vi "Sscard屏幕.vi"() -> ()   [LabVIEW 2015]
uses:
  Controls Type/square.ctl
  <userlib>/QMH/Message Queue/Support/Message Cluster.ctl
  Global control/global-1.vi
  Global control/global-opc.vi
  <userlib>/QMH/Message Queue/Support/Enqueue Message (Single).vi
  <userlib>/QMH/Message Queue/Support/Enqueue Message (Array).vi
  Global control/global-2.vi
  <userlib>/QMH/User Event - Stop/User Event - Stop.lvlib
  <userlib>/QMH/Message Queue/Message Queue.lvlib
panel:
  in  "70":T1
  in  "60":T1
  out "整流柜远程/本地":enum16{"零位", "本地", "远方"}(ring)
  out "直流继保远程/本地":enum16{"零位", "本地", "远方"}(ring)
  out "上网柜远程/本地":enum16{"零位", "本地", "远方"}(ring)
  out "负极柜远程/本地":enum16{"零位", "本地", "远方"}(ring)
  out "馈线柜远程/本地":enum16{"零位", "本地", "远方"}(ring)
  out "进线柜远程/本地":enum16{"零位", "本地", "远方"}(ring)
  out "整流柜远程/本地":enum16{"零位", "本地", "远方"}(ring)
  out "拉伸界面":bool
  in  "HostThread":variant
  in  "Exit":bool
  out "安全运行":string caption="天"
  out "时间":string="14 : 47 : 23" caption="天"
  out "星期":string caption="星\n期"
  out "日":string caption="天"
  out "月":string caption="天"
  out "年":string caption="天"
  in  "405":T1
  in  "406":T1
  in  "407":T1
  in  "445":T1
  in  "213":T1
  in  "211":T1
  in  "90":T1
  in  "214":T1
  in  "212":T1
  in  "402":T1
  in  "401":T1
  in  "241":T1
  in  "226":T1
  in  "202":T1
  in  "245":T1
  in  "231":T1
  in  "237":bool
  in  "236":bool
  in  "225":bool
  in  "201":bool
  in  "2120":bool
  in  "2130":bool
  in  "2110":bool
  in  "2140":bool
  in  "2121":bool
  in  "2124":bool
  in  "2141":bool
  in  "2113":bool
  in  "2111":bool
  in  "2131":bool
  in  "404":bool
  in  "75":bool
  in  "65":bool
  in  "2451":bool
  in  "241-7":bool
  in  "231-7":bool
  in  "237-7":bool
  in  "236-7":bool
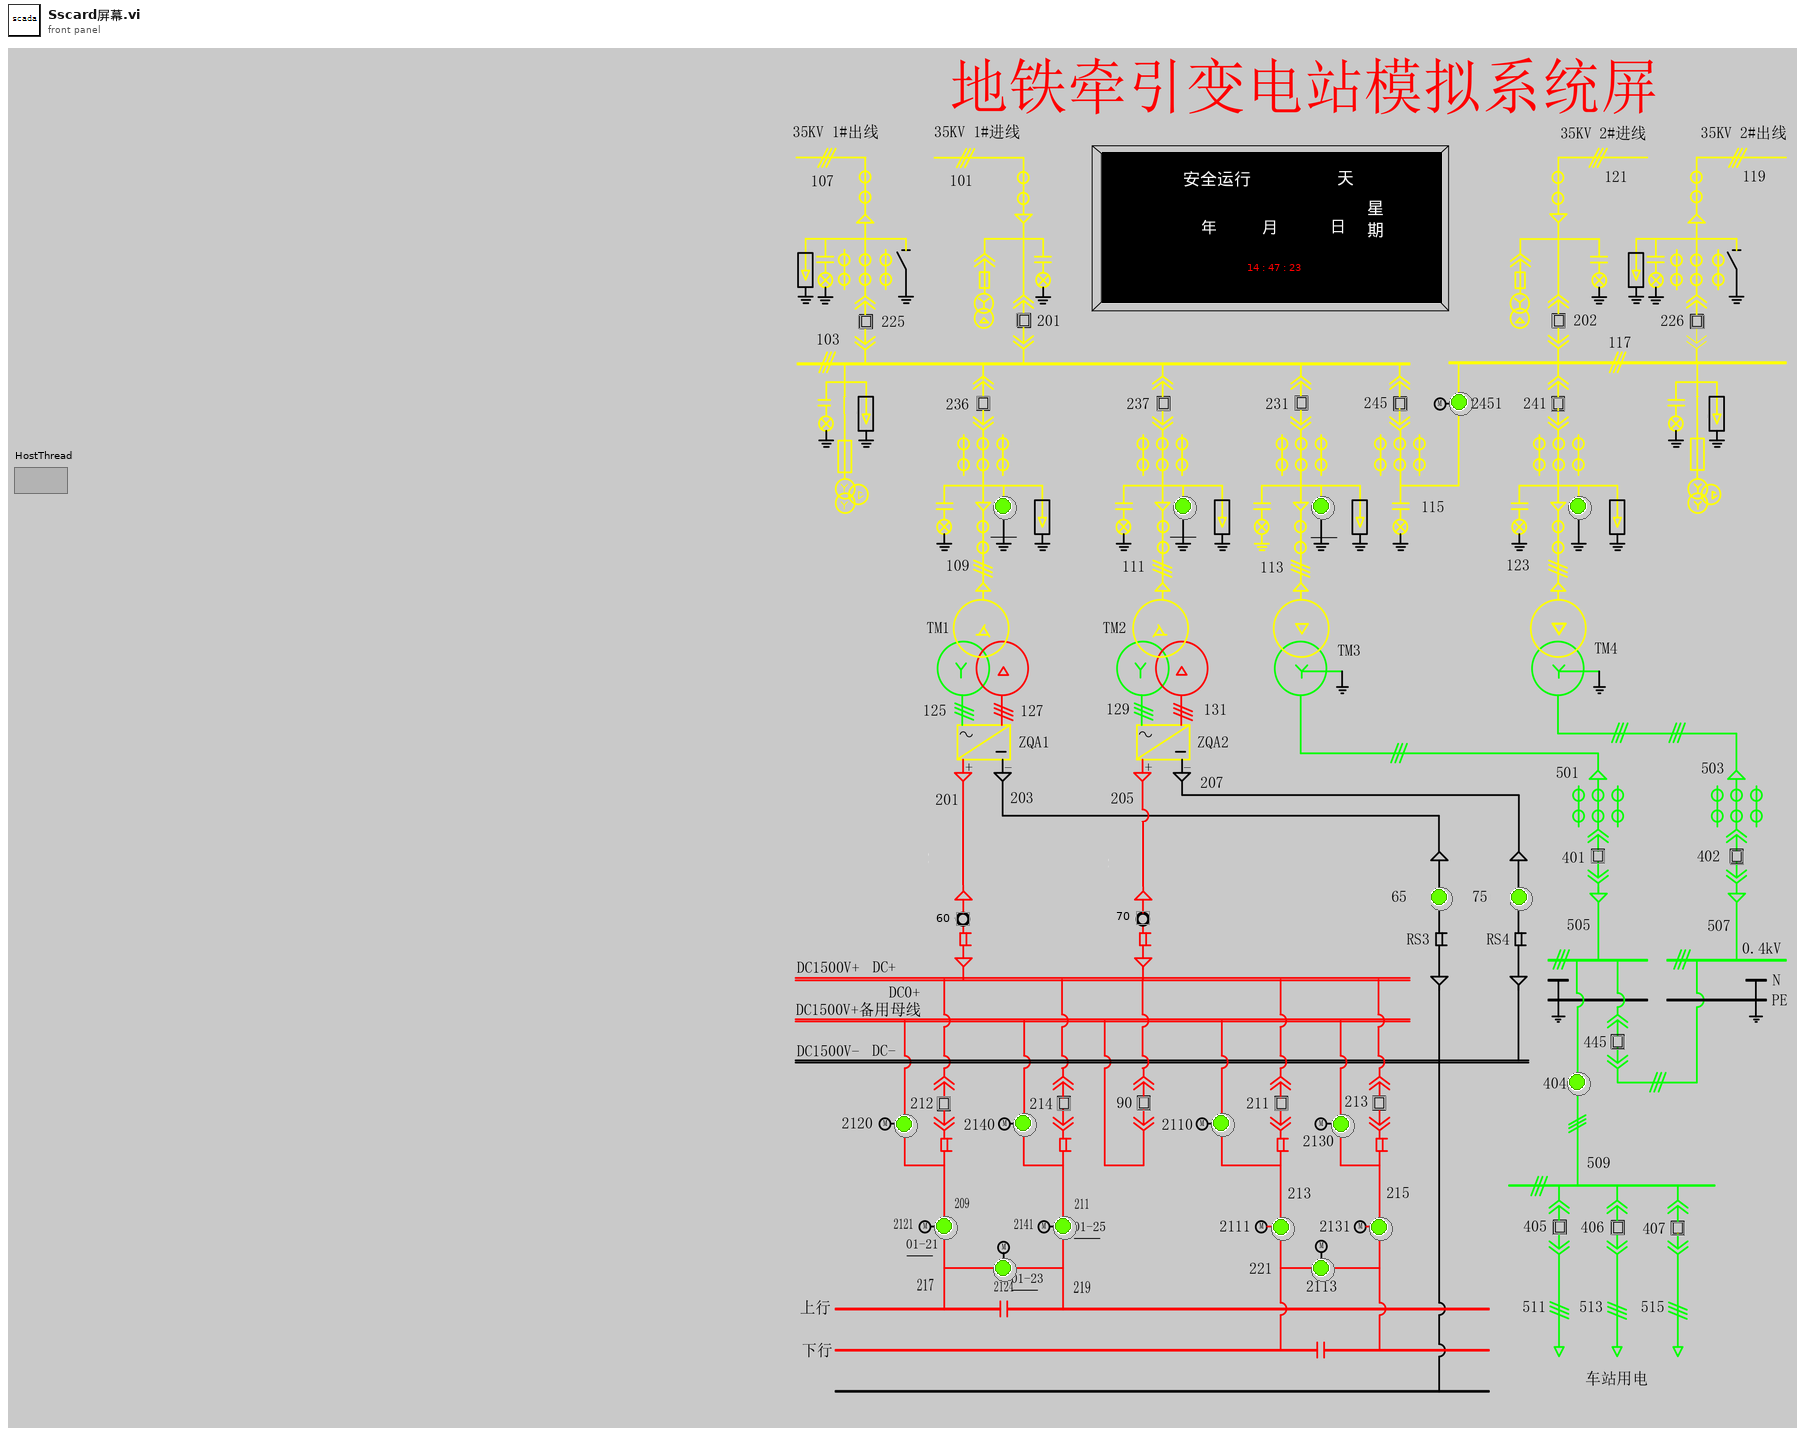
[diagram p1: front panel]
types:
  T1 = typedef "square.ctl" = bool
  T2 = cluster{"Controls":cluster{"Exit":refnum<vi>}, "Thread":cluster{"ThisQ":string, "ThisVI":refnum<vi>, "HostQ":string, "HostRef":refnum<vi>, "SlavesQ":string[], "SlavesRef":refnum<vi>[]}, "Data":cluster{"Replace":bool}, "User":cluster{"Name":string}, "远程本地":cluster{"整流柜远程/本地":enum16{"零位", "本地", "远方"}, "进线柜远程/本地":enum16{"零位", "本地", "远方"}, "馈线柜远程/本地":enum16{"零位", "本地", "远方"}, "负极柜远程/本地":enum16{"零位", "本地", "远方"}, "上网柜远程/本地":enum16{"零位", "本地", "远方"}, "直流继保远程/本地":enum16{"零位", "本地", "远方"}}, "1-1":cluster{"225":refnum<vi>, "201":refnum<vi>, "202":refnum<vi>, "226":refnum<vi>, "236":refnum<vi>, "236-7":refnum<vi>, "237":refnum<vi>, "237-7":refnum<vi>, "231":refnum<vi>, "231-7":refnum<vi>, "245":refnum<vi>, "2451":refnum<vi>, "241":refnum<vi>, "241-7":refnum<vi>}, "1-2":cluster{"60":refnum<vi>, "70":refnum<vi>, "2120":refnum<vi>, "212":refnum<vi>, "2121":refnum<vi>, "2124":refnum<vi>, "214":refnum<vi>, "2140":refnum<vi>, "2141":refnum<vi>, "90":refnum<vi>, "2110":refnum<vi>, "211":refnum<vi>, "2111":refnum<vi>, "2113":refnum<vi>}, "2":cluster{"65":refnum<vi>, "75":refnum<vi>, "401":refnum<vi>, "402":refnum<vi>, "445":refnum<vi>, "404":refnum<vi>, "213":refnum<vi>, "2130":refnum<vi>, "2131":refnum<vi>, "405":refnum<vi>, "406":refnum<vi>, "407":refnum<vi>}, "Message Queue":refnum<queue>}
  T3 = cluster{"225":bool, "201":bool, "202":bool, "226":bool, "236":bool, "236-7":bool, "237":bool, "237-7":bool, "231":bool, "231-7":bool, "245":bool, "2451":bool, "241":bool, "241-7":bool, "备用1":bool, "备用2":bool}
  T4 = cluster{"60":T1, "70":T1, "2120":bool, "212":T1, "2121":bool, "2124":bool, "214":T1, "2140":bool, "2141":bool, "90":T1, "2110":bool, "211":T1, "2111":bool, "2113":bool, "2113":bool, "2113":bool}
  T5 = cluster{"65":bool, "75":bool, "401":T1, "402":T1, "445":T1, "404":bool, "213":T1, "2130":bool, "2131":bool, "405":T1, "406":T1, "407":T1, "407":T1, "407":T1, "407":T1, "407":T1}
  T6 = cluster{"toHMI刀开关合—状态":bool, "toHMI刀开关分—状态":bool, "toHMI刀开关合按钮":bool, "toHMI刀开关分按钮":bool, "toHMI远程":bool, "toHMI本地":bool, "toHMI正常运行":bool, "toHMI设备准备好":bool, "toHMI设备异常":bool, "toHMI刀闸合—动作":bool, "toHMI刀闸分—动作":bool, "toHMI接触轨有压":bool, "刀开关合闸控制":bool, "刀开关分闸控制":bool}
  T7 = cluster{"toHMI正常运行":bool, "toHMI设备准备好":bool, "toHMI设备异常":bool, "toHMI高断分—状态":bool, "toHMI高断合—状态":bool, "toHMI继保故障信号":bool, "toHMI远方":bool, "toHMI本地":bool, "toHMI旁路合闸—按钮":bool, "toHMI旁路分闸—按钮":bool, "toHMI允许高断合闸—状态":bool, "toHMI旁路合分闸—状态":bool, "1500V电压输出":u32, "高断储能控制":bool, "旁路合闸控制":bool, "旁路分闸控制":bool}
  T8 = cluster{"整流柜远程/本地":enum16{"零位", "本地", "远方"}, "进线柜远程/本地":enum16{"零位", "本地", "远方"}, "馈线柜远程/本地":enum16{"零位", "本地", "远方"}, "负极柜远程/本地":enum16{"零位", "本地", "远方"}, "上网柜远程/本地":enum16{"零位", "本地", "远方"}, "直流继保远程/本地":enum16{"零位", "本地", "远方"}}
  T9 = enum8{"Enabled", "Disabled", "Disabled and Grayed Out"}
  T10 = cluster{"1-1":cluster{"225":refnum<vi>, "201":refnum<vi>, "202":refnum<vi>, "226":refnum<vi>, "236":refnum<vi>, "236-7":refnum<vi>, "237":refnum<vi>, "237-7":refnum<vi>, "231":refnum<vi>, "231-7":refnum<vi>, "245":refnum<vi>, "2451":refnum<vi>, "241":refnum<vi>, "241-7":refnum<vi>}, "1-2":cluster{"60":refnum<vi>, "70":refnum<vi>, "2120":refnum<vi>, "212":refnum<vi>, "2121":refnum<vi>, "2124":refnum<vi>, "214":refnum<vi>, "2140":refnum<vi>, "2141":refnum<vi>, "90":refnum<vi>, "2110":refnum<vi>, "211":refnum<vi>, "2111":refnum<vi>, "2113":refnum<vi>}, "2":cluster{"65":refnum<vi>, "75":refnum<vi>, "401":refnum<vi>, "402":refnum<vi>, "445":refnum<vi>, "404":refnum<vi>, "213":refnum<vi>, "2130":refnum<vi>, "2131":refnum<vi>, "405":refnum<vi>, "406":refnum<vi>, "407":refnum<vi>}}
  T11 = cluster{"225":refnum<vi>, "201":refnum<vi>, "202":refnum<vi>, "226":refnum<vi>, "236":refnum<vi>, "236-7":refnum<vi>, "237":refnum<vi>, "237-7":refnum<vi>, "231":refnum<vi>, "231-7":refnum<vi>, "245":refnum<vi>, "2451":refnum<vi>, "241":refnum<vi>, "241-7":refnum<vi>}
  T12 = cluster{"60":refnum<vi>, "70":refnum<vi>, "2120":refnum<vi>, "212":refnum<vi>, "2121":refnum<vi>, "2124":refnum<vi>, "214":refnum<vi>, "2140":refnum<vi>, "2141":refnum<vi>, "90":refnum<vi>, "2110":refnum<vi>, "211":refnum<vi>, "2111":refnum<vi>, "2113":refnum<vi>}
  T13 = cluster{"65":refnum<vi>, "75":refnum<vi>, "401":refnum<vi>, "402":refnum<vi>, "445":refnum<vi>, "404":refnum<vi>, "213":refnum<vi>, "2130":refnum<vi>, "2131":refnum<vi>, "405":refnum<vi>, "406":refnum<vi>, "407":refnum<vi>}
  T14 = cluster{"toHMI正常运行":bool, "toHMI异常跳闸":bool, "toHMI远程":bool, "toHMI模拟中压合闸—按钮":bool, "toHMI负极柜故障报警":bool, "toHMI正极柜故障报警":bool, "toHMI馈线柜故障报警":bool, "toHMI上网柜故障报警":bool, "toHMI整流柜故障报警":bool, "toHMI压敏快熔故障":bool, "toHMI整流柜跳闸":bool, "toHMI整流柜合闸—状态":bool, "直流电流输出":u32, "直流220V电压输出":u32, "380电压输入":u32, "模拟中压合闸控制":bool, "toHMI本地":bool}
  T15 = cluster{"toHMI正常运行":bool, "toHMI设备准备好":bool, "toHMI设备异常":bool, "toHMI刀开关分—状态":bool, "toHMI刀开关合—状态":bool, "toHMI框架电流故障":bool, "toHMI框架电压故障":bool, "toHMII段电压故障":bool, "toHMIII段电压故障":bool, "toHMI装置故障":bool, "toHMIMCB故障":bool, "toHMI刀开关合—完成":bool, "toHMI复位按钮":bool, "toHMI远程":bool, "toHMI本地":bool, "模拟电流框架故障控制":bool, "模拟电压框架故障控制":bool, "模拟I段电压故障控制":bool, "模拟II段电压故障控制":bool, "故障复位控制":bool}
  T16 = cluster{"直接合闸":bool, "分闸复位":bool, "带测合闸":bool, "MCB故障":bool, "断路器合闸反馈信号":bool, "ED储能":bool, "应急分闸":bool, "断路器分闸反馈信号":bool, "远程控制":bool, "就地控制":bool, "试验位置":bool, "工作位置":bool, "带测接触器":bool, "本站框架":bool, "邻站过流":bool, "邻站框架":bool}
  T17 = cluster{"toHMI正常运行":bool, "toHMI设备准备好":bool, "toHMI设备异常":bool, "toHMI刀开关合—状态":bool, "toHMI刀开关分—状态":bool, "toHMI刀开关合按钮":bool, "toHMI刀开关分按钮":bool, "toHMI复位按钮":bool, "toHMI远程":bool, "toHMI本地":bool, "toHMI刀闸合—动作":bool, "toHMI刀闸分—动作":bool, "刀开关合闸控制":bool, "刀开关分闸控制":bool, "故障复位控制":bool}
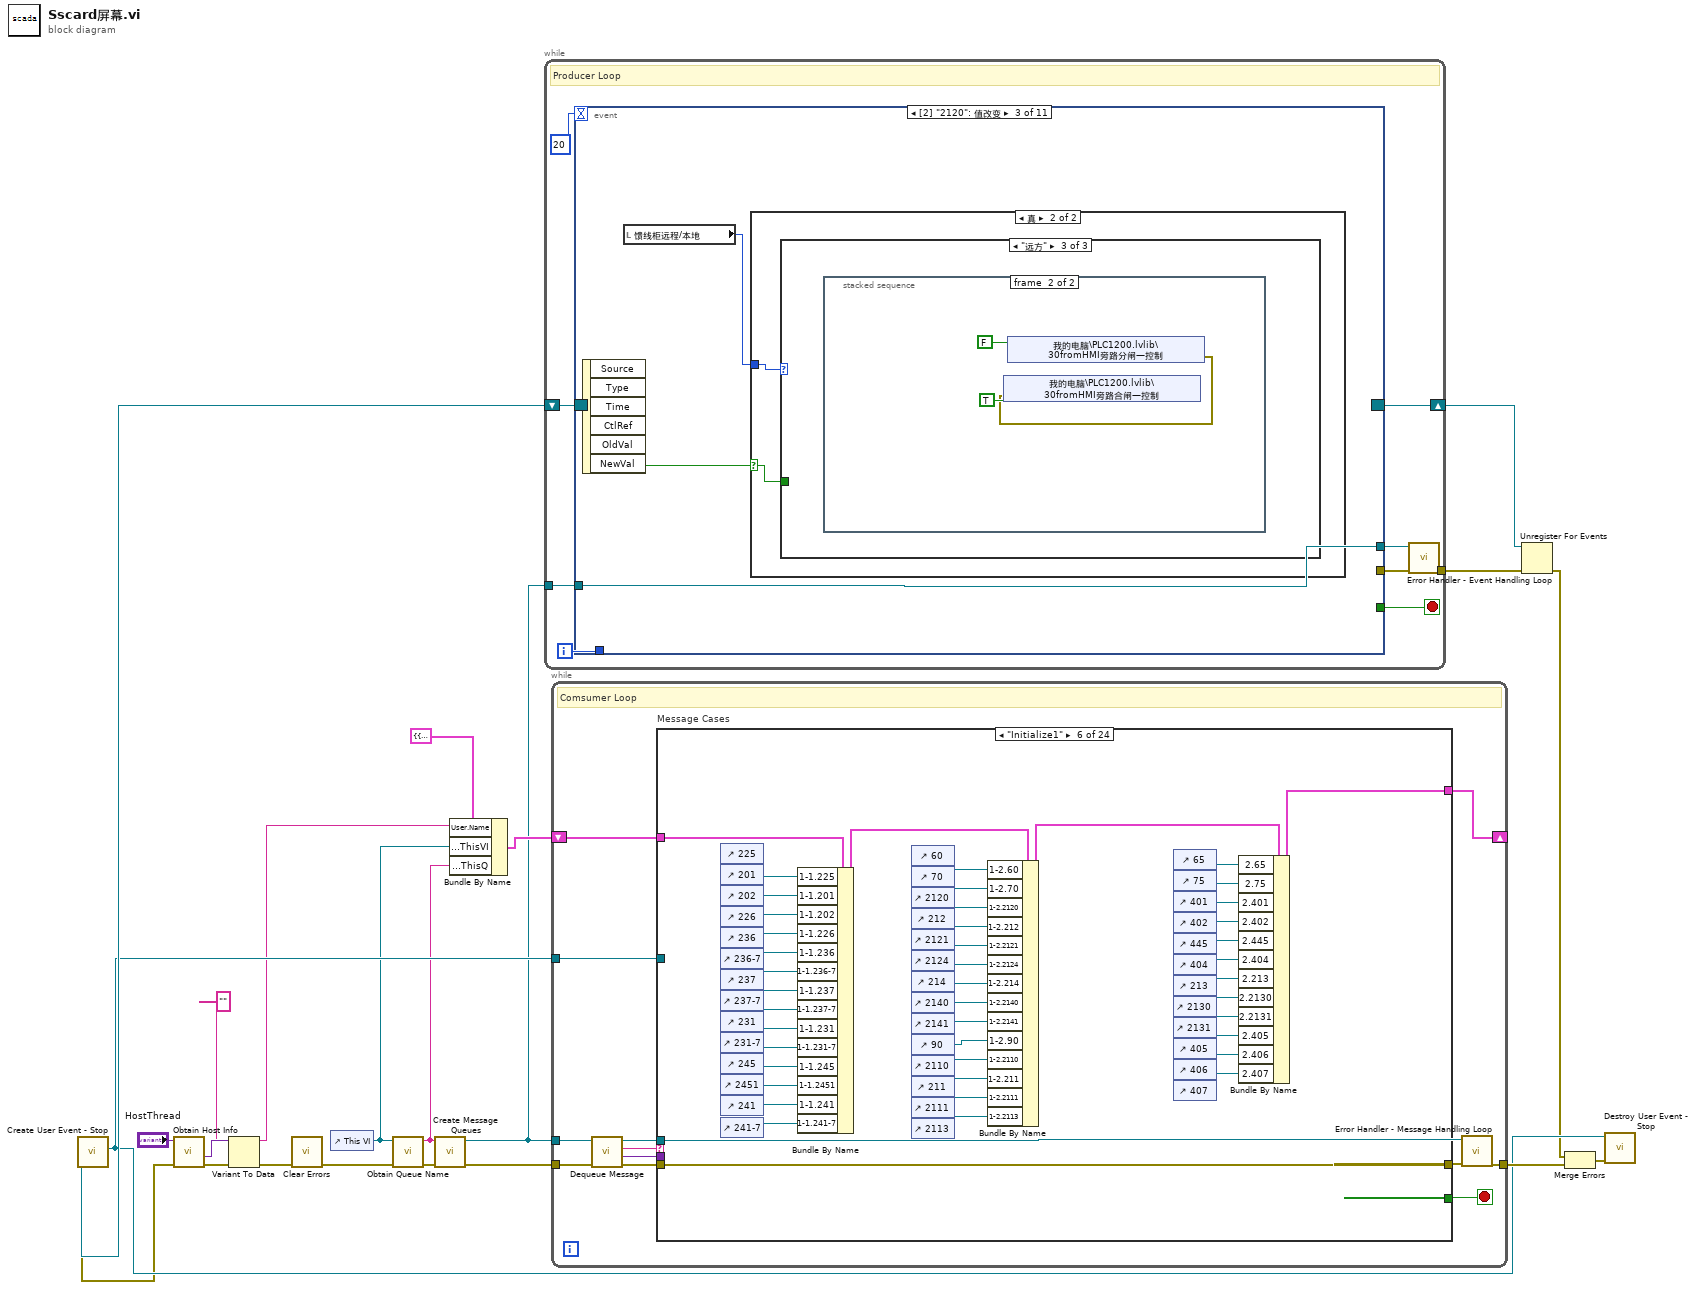
[diagram p0: block diagram]
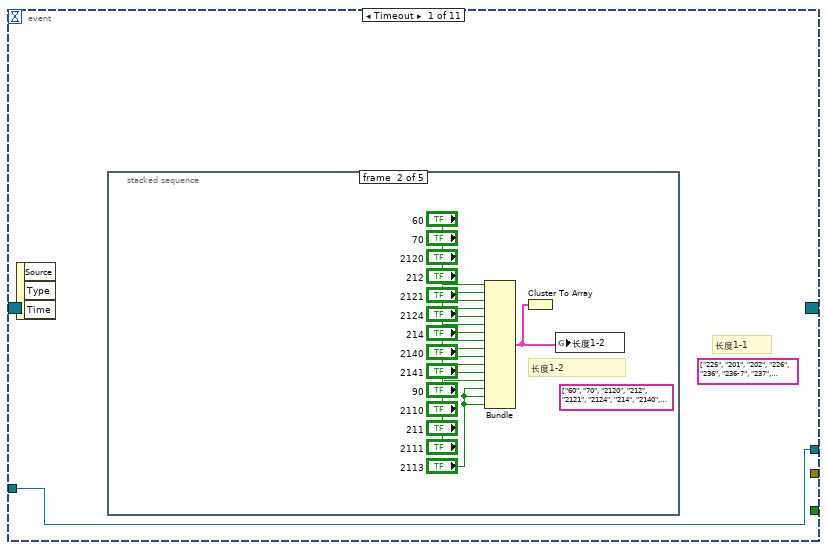
[diagram p2: hidden frame]
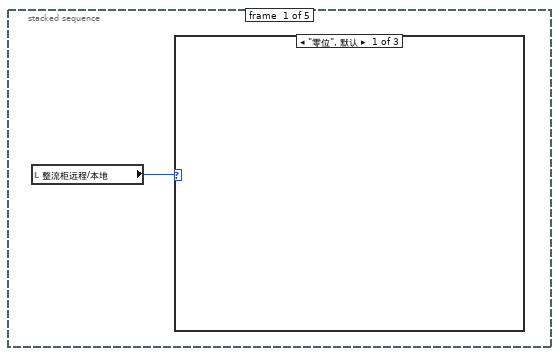
[diagram p3: hidden frame]
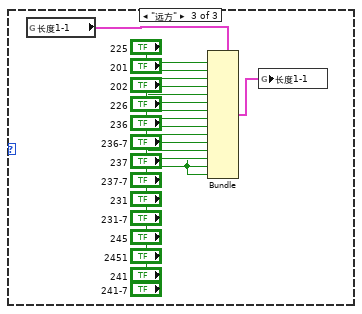
[diagram p5: hidden frame]
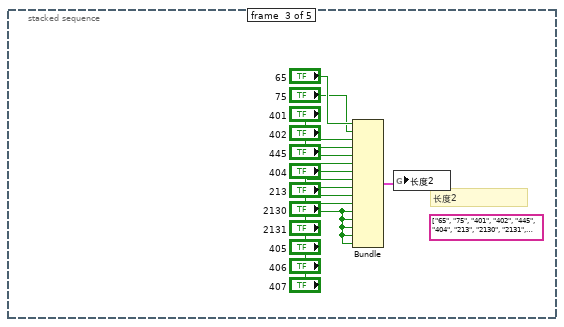
[diagram p6: hidden frame]
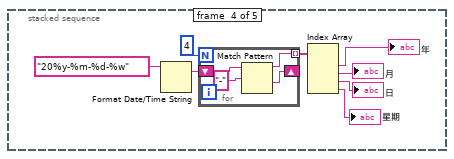
[diagram p7: hidden frame]
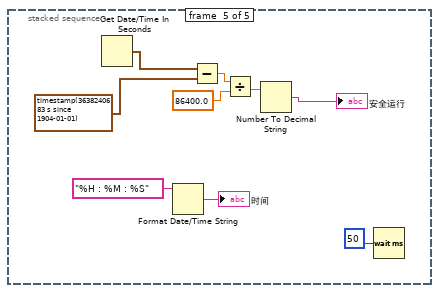
[diagram p8: hidden frame]
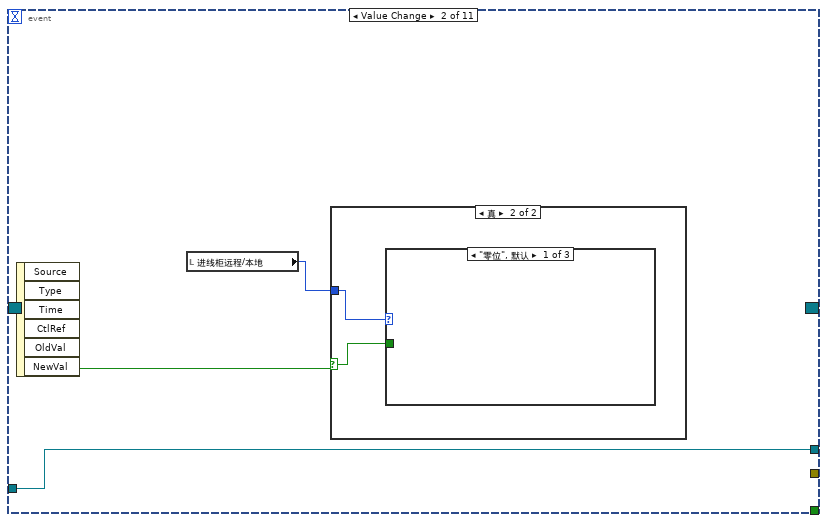
[diagram p9: hidden frame]
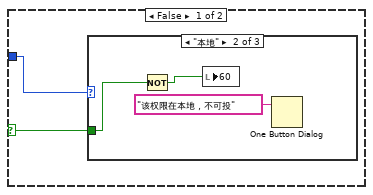
[diagram p10: hidden frame]
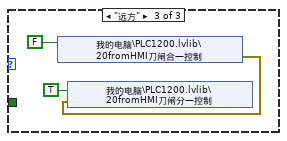
[diagram p12: hidden frame]
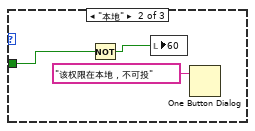
[diagram p13: hidden frame]
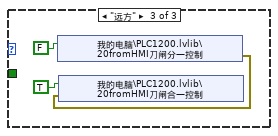
[diagram p14: hidden frame]
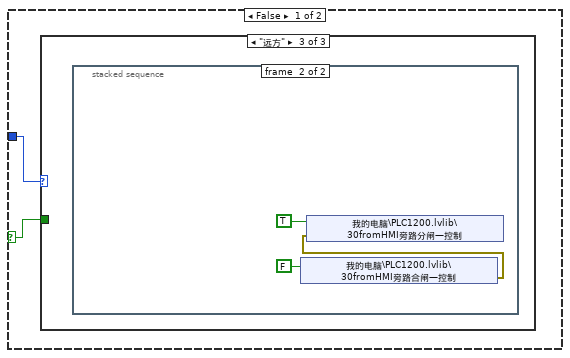
[diagram p15: hidden frame]
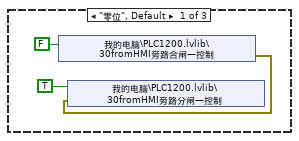
[diagram p16: hidden frame]
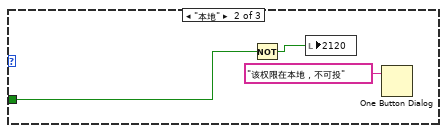
[diagram p17: hidden frame]
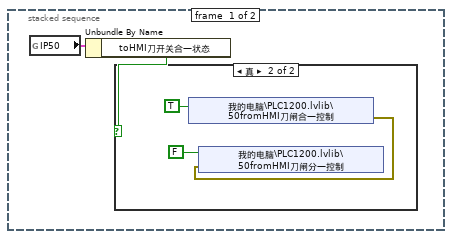
[diagram p18: hidden frame]
diagram:
  n1 = call <userlib>:"Create User Event - Stop.vi"() -> ("error out"=w9:errorcluster, "User Event - Stop"=w18:refnum<user-event>, "Stop Event Registration Refnum"=w20:refnum<event-registration>)  [unwired: 9 in]
  n2 = call <userlib>:"Obtain Host Info.vi"("error in (no error)"=w9, "HostThread"="HostThread") -> ("error out"=w6:errorcluster, "Data"=w5:variant)  [unwired: 6 in, 2 out]
  n3 = Variant To Data(error in=w6, type="", Variant=w5) -> (data=w1:string, error out=w3:errorcluster)
  n4 = call <vilib>:"Clear Errors.vi"("error in (no error)"=w3) -> ("error out"=w2:errorcluster)  [unwired: 5 in, 1 out]
  n5 = control-ref of="This VI"() -> (w11:refnum<vi>)
  n6 = call <userlib>:"Obtain Queue Name.vi"("error in (no error)"=w2, "VI Refnum"=w11) -> ("error out"=w14:errorcluster, "ViName"=w10:string)  [unwired: 8 in]
  n7 = call <userlib>:"Create Message Queues.vi"("error in (no error)"=w14, "name (unnamed)"=w10) -> ("error out"=w22:errorcluster, "QueueHandler"=w7:refnum<queue>)  [unwired: 8 in]
  n8 = Bundle By Name(cluster=T2 {"Controls"={"Exit"=refnum}, "Thread"={"ThisQ"="", "ThisVI"=refnum, "HostQ"="", "HostRef"=refnum, "SlavesQ"=[], "SlavesRef"=[]}, "Data"={"Replace"=FALSE}, "User"={"Name"=""}, "远程本地"={"整流柜远程/本地"=enum."零位", "进线柜远程/本地"=enum."零位", "馈线柜远程/本地"=enum."零位", "负极柜远程/本地"=enum."零位", "上网柜远程/本地"=enum."零位", "直流继保远程/本地"=enum."零位"}, "1-1"={"225"=refnum, "201"=refnum, "202"=refnum, "226"=refnum, "236"=refnum, "236-7"=refnum, "237"=refnum, "237-7"=refnum, "231"=refnum, "231-7"=refnum, "245"=refnum, "2451"=refnum, "241"=refnum, "241-7"=refnum}, "1-2"={"60"=refnum, "70"=refnum, "2120"=refnum, "212"=refnum, "2121"=refnum, "2124"=refnum, "214"=refnum, "2140"=refnum, "2141"=refnum, "90"=refnum, "2110"=refnum, "211"=refnum, "2111"=refnum, "2113"=refnum}, "2"={"65"=refnum, "75"=refnum, "401"=refnum, "402"=refnum, "445"=refnum, "404"=refnum, "213"=refnum, "2130"=refnum, "2131"=refnum, "405"=refnum, "406"=refnum, "407"=refnum}, "Message Queue"=refnum} ("Data Cluster"), "User.Name"=w1, "Thread.ThisVI"=w11, "Thread.ThisQ"=w10) -> (w12:T2)
  n9 = while {
    tunnel: w7 -> [w31]
    shift-right: [w29] -> w16
    shift-left: w20 -> [w30]
    tunnel: [w25] -> w15
    i -> [w23]
    stop <- w27 stop-if-true
    # "Producer Loop"
    n10 = event shown="[2] \"2120\": 值改变" {
      selector: w30 -> [_ _ _ _ _ _ _ _ _ _ _]
      dyn-events: [_ _ _ _ _ _ _ _ _ _ _] -> w29
      timeout: 20 -> [_ _ _ _ _ _ _ _ _ _ _]
      tunnel: [_ _ _ _ _ _ _ _ _ TRUE ("Discard?") _] -> w27
      tunnel: w31 -> [w32 w101 w119 w160 w186 w242 w282 w329 w331 w333 w338]
      tunnel: [_ _ _ _ _ _ _ w328 _ _ w336] -> w28
      tunnel: [w32 w101 w119 w160 w186 w242 w282 w327 w331 w333 w337] -> w26
      tunnel: w23 -> [_ _ _ _ _ _ _ _ _ _ _]
      event Timeout {
        (unwired) string[] ["225", "201", "202", "226", "236", "236-7", "237", "237-7", "231", "231-7", "245", "2451", "241", "241-7"]
        # "长度1-1"
        # "Add circle collection here; And according to the different signal, we should build the \"Choose Box\"."
        n11 = event-data() -> ()  [unwired: 1 in, 3 out]
        n12 = stacked-sequence {
          frame #0 {
            n13 = local read "整流柜远程/本地"() -> (w33:enum16{"零位", "本地", "远方"})
            n14 = case shown="\"零位\", 默认" w33 {
              frame "零位", Default {
              }
              frame "本地" {
              }
              frame "远方" {
                n15 = global read "global-1.vi" "长度1-1"() -> (w36:T3)
                n16 = Bundle(cluster=w36, "225"="225", "201"="201", "202"="202", "226"="226", "236"="236", "236-7"="236-7", "237"="237", "237-7"="237-7", "231"="231", "231-7"="231-7", "245"="245", "2451"="2451", "241"="241", "241-7"="241-7", "备用1"="241-7", "备用2"="241-7") -> (w34:T3)
                n17 = global write "global-1.vi" "长度1-1"(w34) -> ()
              }
            }
          }
          frame #1 {
            (unwired) string[] ["60", "70", "2120", "212", "2121", "2124", "214", "2140", "2141", "90", "2110", "211", "2111", "2113"]
            # "长度1-2"
            n18 = Bundle("60"="60", "70"="70", "2120"="2120", "212"="212", "2121"="2121", "2124"="2124", "214"="214", "2140"="2140", "2141"="2141", "90"="90", "2110"="2110", "211"="211", "2111"="2111", "2113"="2113", "2113"="2113", "2113"="2113") -> (w50:T4)  [unwired: 1 in]
            n19 = Cluster To Array(cluster=w50) -> ()  [unwired: 1 out]
            n20 = global write "global-1.vi" "长度1-2"(w50) -> ()
          }
          frame #2 {
            (unwired) string[] ["65", "75", "401", "402", "445", "404", "213", "2130", "2131", "405", "406", "407"]
            # "长度2"
            n21 = Bundle("65"="65", "75"="75", "401"="401", "402"="402", "445"="445", "404"="404", "213"="213", "2130"="2130", "2131"="2131", "405"="405", "406"="406", "407"="407", "407"="407", "407"="407", "407"="407", "407"="407") -> (w65:T5)  [unwired: 1 in]
            n22 = global write "global-1.vi" "长度2"(w65) -> ()
          }
          frame #3 {
            n23 = Format Date/Time String(time format string (%c)="20%y-%m-%d-%w" ("时间格式字符串(%c)")) -> (date/time string=w81:string)  [unwired: 2 in]
            n24 = for {
              N: 4 -> [_]
              shift-right: [w87] -> _
              shift-left: w81 -> [w88]
              tunnel: [w86] -> w83 mode=indexing
              n25 = Match Pattern(string=w88, regular expression="-" ("正则表达式")) -> (before substring=w86:string, after substring=w87:string)  [unwired: 1 in, 2 out]
            }
            n26 = Index Array(array=w83) -> (element #1=→"年":string, element #2=→"月":string, element #3=→"日":string, element #4=→"星期":string)  [unwired: 4 in]
          }
          frame #4 {
            n27 = Get Date/Time In Seconds() -> (seconds since 1Jan1904=w96:timestamp)
            n28 = Format Date/Time String(time format string (%c)="%H : %M : %S" ("时间格式字符串(%c)")) -> (date/time string=→"时间":string)  [unwired: 2 in]
            n29 = Subtract(x=w96, y=timestamp(3638240683.009 s since 1904-01-01) ("时间标识")) -> (x-y=w94:dbl)
            n30 = Divide(x=w94, y=86400.0) -> (x/y=w92:dbl)
            n31 = Number To Decimal String(number=w92) -> (decimal integer string=→"安全运行":string)  [unwired: 1 in]
            n32 = Wait (ms)(milliseconds to wait=u32 50 ("等待时间（毫秒）")) -> ()  [unwired: 1 out]
          }
        }
      }
      event Value Change {
        n33 = event-data() -> ("NewVal"=w100:T1)  [unwired: 1 in, 5 out]
        n34 = local read "进线柜远程/本地"() -> (w99:enum16{"零位", "本地", "远方"})
        n35 = case shown="真" w100 {
          selector: w100 -> [w103 w111]
          tunnel: w99 -> [w102 w110]
          frame False {
            n36 = case shown="\"本地\"" w102 {
              tunnel: w103 -> [_ w104 _]
              frame "零位", Default {
              }
              frame "本地" {
                n37 = Not(x=w104) -> (.not. x?=w105:bool)
                n38 = local write "60"(w105) -> ()
                n39 = One Button Dialog(message="该权限在本地，不可投" ("消息")) -> ()  [unwired: 1 in, 1 out]
              }
              frame "远方" {
                n40 = shared-variable "我的电脑\\PLC1200.lvlib\\20fromHMI刀闸合—控制"(FALSE) -> (error out=w108:errorcluster)  [unwired: 1 in]
                n41 = shared-variable "我的电脑\\PLC1200.lvlib\\20fromHMI刀闸分—控制"(TRUE, error in=w108) -> ()  [unwired: 1 out]
              }
            }
          }
          frame True {
            n42 = case shown="\"零位\", 默认" w110 {
              tunnel: w111 -> [_ w113 _]
              frame "零位", Default {
              }
              frame "本地" {
                n43 = Not(x=w113) -> (.not. x?=w112:bool)
                n44 = local write "60"(w112) -> ()
                n45 = One Button Dialog(message="该权限在本地，不可投" ("消息")) -> ()  [unwired: 1 in, 1 out]
              }
              frame "远方" {
                n46 = shared-variable "我的电脑\\PLC1200.lvlib\\20fromHMI刀闸分—控制"(FALSE) -> (error out=w116:errorcluster)  [unwired: 1 in]
                n47 = shared-variable "我的电脑\\PLC1200.lvlib\\20fromHMI刀闸合—控制"(TRUE, error in=w116) -> ()  [unwired: 1 out]
              }
            }
          }
        }
      }
      event "2120": Value Change {
        n48 = event-data() -> ("NewVal"=w118:bool)  [unwired: 1 in, 5 out]
        n49 = local read "馈线柜远程/本地"() -> (w120:enum16{"零位", "本地", "远方"})
        n50 = case shown="真" w118 {
          selector: w118 -> [w122 w138]
          tunnel: w120 -> [w121 w137]
          frame False {
            n51 = case shown="\"远方\"" w121 {
              tunnel: w122 -> [_ w126 _]
              frame "零位", Default {
                n52 = shared-variable "我的电脑\\PLC1200.lvlib\\30fromHMI旁路合闸—控制"(FALSE) -> (error out=w123:errorcluster)  [unwired: 1 in]
                n53 = shared-variable "我的电脑\\PLC1200.lvlib\\30fromHMI旁路分闸—控制"(TRUE, error in=w123) -> ()  [unwired: 1 out]
              }
              frame "本地" {
                n54 = Not(x=w126) -> (.not. x?=w127:bool)
                n55 = local write "2120"(w127) -> ()
                n56 = One Button Dialog(message="该权限在本地，不可投" ("消息")) -> ()  [unwired: 1 in, 1 out]
              }
              frame "远方" {
                n57 = stacked-sequence {
                  frame #0 {
                    n58 = global read "global-opc.vi" "IP50"() -> (w130:T6)
                    n59 = Unbundle By Name(w130) -> ("toHMI刀开关合—状态"=w129:bool)
                    n60 = case shown="真" w129 {
                      frame False {
                      }
                      frame True {
                        n61 = shared-variable "我的电脑\\PLC1200.lvlib\\50fromHMI刀闸合—控制"(TRUE) -> (error out=w131:errorcluster)  [unwired: 1 in]
                        n62 = shared-variable "我的电脑\\PLC1200.lvlib\\50fromHMI刀闸分—控制"(FALSE, error in=w131) -> ()  [unwired: 1 out]
                      }
                    }
                  }
                  frame #1 {
                    n63 = shared-variable "我的电脑\\PLC1200.lvlib\\30fromHMI旁路合闸—控制"(FALSE) -> (error out=w134:errorcluster)  [unwired: 1 in]
                    n64 = shared-variable "我的电脑\\PLC1200.lvlib\\30fromHMI旁路分闸—控制"(TRUE, error in=w134) -> ()  [unwired: 1 out]
                  }
                }
              }
            }
          }
          frame True {
            n65 = case shown="\"远方\"" w137 {
              tunnel: w138 -> [_ w140 _]
              frame "零位", Default {
              }
              frame "本地" {
                n66 = Not(x=w140) -> (.not. x?=w139:bool)
                n67 = local write "2120"(w139) -> ()
                n68 = One Button Dialog(message="该权限在本地，不可投" ("消息")) -> ()  [unwired: 1 in, 1 out]
              }
              frame "远方" {
                n69 = stacked-sequence {
                  frame #0 {
                    n70 = stacked-sequence {
                      frame #0 {
                        n71 = global read "global-opc.vi" "IP30"() -> (w143:T7)
                        n72 = Unbundle By Name(w143) -> ("toHMI高断合—状态"=w142:bool)
                        n73 = case shown="假" w142 {
                          frame False {
                          }
                          frame True {
                            n74 = call <userlib>:"Obtain Message Queue.vi"("name (unnamed)"="继保.vi") -> ("Message Queue"=w149:refnum<queue>)  [unwired: 9 in, 1 out]
                            n75 = Bundle(u16 256, TRUE) -> (w145:cluster{u16, bool})  [unwired: 1 in]
                            n76 = call-poly <userlib>:"Enqueue Message.vi"("Message Data"=w145, "Message"="遥控", "Message Queue"=w149) -> ()  [unwired: 7 in, 2 out]
                          }
                        }
                      }
                      frame #1 {
                        n77 = global read "global-opc.vi" "IP50"() -> (w151:T6)
                        n78 = Unbundle By Name(w151) -> ("toHMI刀开关合—状态"=w150:bool)
                        n79 = case shown="真" w150 {
                          frame False {
                          }
                          frame True {
                            n80 = shared-variable "我的电脑\\PLC1200.lvlib\\50fromHMI刀闸合—控制"(TRUE) -> (error out=w152:errorcluster)  [unwired: 1 in]
                            n81 = shared-variable "我的电脑\\PLC1200.lvlib\\50fromHMI刀闸分—控制"(FALSE, error in=w152) -> ()  [unwired: 1 out]
                          }
                        }
                      }
                    }
                  }
                  frame #1 {
                    n82 = shared-variable "我的电脑\\PLC1200.lvlib\\30fromHMI旁路分闸—控制"(FALSE) -> (error out=w155:errorcluster)  [unwired: 1 in]
                    n83 = shared-variable "我的电脑\\PLC1200.lvlib\\30fromHMI旁路合闸—控制"(TRUE, error in=w155) -> ()  [unwired: 1 out]
                  }
                }
              }
            }
          }
        }
      }
      event "2121": Value Change {
        n84 = event-data() -> ("NewVal"=w158:bool)  [unwired: 1 in, 5 out]
        n85 = local read "上网柜远程/本地"() -> (w159:enum16{"零位", "本地", "远方"})
        n86 = case shown="真" w158 {
          selector: w158 -> [w162 w173]
          tunnel: w159 -> [w161 w172]
          frame False {
            n87 = case shown="\"本地\"" w161 {
              tunnel: w162 -> [_ w166 _]
              frame "零位", Default {
                n88 = shared-variable "我的电脑\\PLC1200.lvlib\\30fromHMI旁路合闸—控制"(FALSE) -> (error out=w163:errorcluster)  [unwired: 1 in]
                n89 = shared-variable "我的电脑\\PLC1200.lvlib\\30fromHMI旁路分闸—控制"(TRUE, error in=w163) -> ()  [unwired: 1 out]
              }
              frame "本地" {
                n90 = Not(x=w166) -> (.not. x?=w167:bool)
                n91 = local write "2121"(w167) -> ()
                n92 = One Button Dialog(message="该权限在本地，不可投" ("消息")) -> ()  [unwired: 1 in, 1 out]
              }
              frame "远方" {
                n93 = shared-variable "我的电脑\\PLC1200.lvlib\\50fromHMI刀闸合—控制"(FALSE) -> (error out=w169:errorcluster)  [unwired: 1 in]
                n94 = shared-variable "我的电脑\\PLC1200.lvlib\\50fromHMI刀闸分—控制"(TRUE, error in=w169) -> ()  [unwired: 1 out]
              }
            }
          }
          frame True {
            n95 = case shown="\"本地\"" w172 {
              tunnel: w173 -> [_ w175 _]
              frame "零位", Default {
              }
              frame "本地" {
                n96 = Not(x=w175) -> (.not. x?=w174:bool)
                n97 = local write "2121"(w174) -> ()
                n98 = One Button Dialog(message="该权限在本地，不可投" ("消息")) -> ()  [unwired: 1 in, 1 out]
              }
              frame "远方" {
                n99 = shared-variable "我的电脑\\PLC1200.lvlib\\50fromHMI刀闸分—控制"(FALSE) -> (error out=w177:errorcluster)  [unwired: 1 in]
                n100 = shared-variable "我的电脑\\PLC1200.lvlib\\50fromHMI刀闸合—控制"(TRUE, error in=w177) -> ()  [unwired: 1 out]
              }
            }
          }
        }
      }
      event Value Change {
        n101 = event-data() -> ("NewVal"=w180:T1)  [unwired: 1 in, 5 out]
        n102 = local read "直流继保远程/本地"() -> (w182:enum16{"零位", "本地", "远方"})
        n103 = global read "global-opc.vi" "IP50"() -> (w185:T6)
        n104 = global read "global-opc.vi" "IP30"() -> (w181:T7)
        n105 = case shown="真" w180 {
          selector: w180 -> [w191 w217]
          tunnel: w182 -> [w190 w216]
          tunnel: ["直流继保远方>高速断路器分闸" ("字符串") "直流继保远方>高速断路器合闸" ("字符串")] -> w183
          tunnel: w185 -> [w188 w214]
          tunnel: w181 -> [w187 w213]
          frame False {
            n106 = case shown="\"远方\"" w190 {
              tunnel: w191 -> [_ w193 _]
              tunnel: w188 -> [_ _ w196]
              tunnel: w187 -> [_ _ w195]
              frame "零位" {
              }
              frame "本地", Default {
                n107 = Not(x=w193) -> (.not. x?=w192:bool)
                n108 = local write "212"(w192) -> ()
                n109 = One Button Dialog(message="该权限在本地，不可投" ("消息")) -> ()  [unwired: 1 in, 1 out]
              }
              frame "远方" {
                n110 = stacked-sequence {
                  tunnel: w196 -> [_ w202 _]
                  tunnel: w195 -> [w198 _ _]
                  frame #0 {
                    n111 = Unbundle By Name(w198) -> ("toHMI旁路合分闸—状态"=w197:bool)
                    n112 = case shown="真" w197 {
                      frame False {
                      }
                      frame True {
                        n113 = shared-variable "我的电脑\\PLC1200.lvlib\\30fromHMI旁路合闸—控制"(FALSE) -> (error out=w201:errorcluster)  [unwired: 1 in]
                        n114 = shared-variable "我的电脑\\PLC1200.lvlib\\30fromHMI旁路分闸—控制"(TRUE, error in=w201) -> ()  [unwired: 1 out]
                      }
                    }
                  }
                  frame #1 {
                    n115 = Unbundle By Name(w202) -> ("toHMI刀开关合—状态"=w203:bool)
                    n116 = case shown="真" w203 {
                      frame False {
                      }
                      frame True {
                        n117 = shared-variable "我的电脑\\PLC1200.lvlib\\50fromHMI刀闸合—控制"(TRUE) -> (error out=w204:errorcluster)  [unwired: 1 in]
                        n118 = shared-variable "我的电脑\\PLC1200.lvlib\\50fromHMI刀闸分—控制"(FALSE, error in=w204) -> ()  [unwired: 1 out]
                      }
                    }
                  }
                  frame #2 {
                    n119 = call <userlib>:"Obtain Message Queue.vi"("name (unnamed)"="继保.vi") -> ("Message Queue"=w212:refnum<queue>)  [unwired: 9 in, 1 out]
                    n120 = Bundle(u16 256, TRUE) -> (w208:cluster{u16, bool})  [unwired: 1 in]
                    n121 = call-poly <userlib>:"Enqueue Message.vi"("Message Data"=w208, "Message"="遥控", "Message Queue"=w212) -> ()  [unwired: 7 in, 2 out]
                  }
                }
              }
            }
          }
          frame True {
            n122 = case shown="\"远方\"" w216 {
              tunnel: w217 -> [_ w218 _]
              tunnel: w214 -> [_ _ w222]
              tunnel: w213 -> [_ _ w221]
              frame "零位" {
              }
              frame "本地", Default {
                n123 = Not(x=w218) -> (.not. x?=w219:bool)
                n124 = local write "212"(w219) -> ()
                n125 = One Button Dialog(message="该权限在本地，不可投" ("消息")) -> ()  [unwired: 1 in, 1 out]
              }
              frame "远方" {
                n126 = stacked-sequence {
                  tunnel: w222 -> [_ _ _]
                  tunnel: w221 -> [w224 _ _]
                  frame #0 {
                    n127 = Unbundle By Name(w224) -> ("toHMI旁路合分闸—状态"=w223:bool)
                    n128 = case shown="真" w223 {
                      frame False {
                      }
                      frame True {
                        n129 = shared-variable "我的电脑\\PLC1200.lvlib\\30fromHMI旁路合闸—控制"(FALSE) -> (error out=w225:errorcluster)  [unwired: 1 in]
                        n130 = shared-variable "我的电脑\\PLC1200.lvlib\\30fromHMI旁路分闸—控制"(TRUE, error in=w225) -> ()  [unwired: 1 out]
                      }
                    }
                  }
                  frame #1 {
                    n131 = global read "global-opc.vi" "IP50"() -> (w229:T6)
                    n132 = Unbundle By Name(w229) -> ("toHMI刀开关合—状态"=w228:bool)
                    n133 = case shown="真" w228 {
                      frame False {
                      }
                      frame True {
                        n134 = shared-variable "我的电脑\\PLC1200.lvlib\\50fromHMI刀闸合—控制"(TRUE) -> (error out=w230:errorcluster)  [unwired: 1 in]
                        n135 = shared-variable "我的电脑\\PLC1200.lvlib\\50fromHMI刀闸分—控制"(FALSE, error in=w230) -> ()  [unwired: 1 out]
                      }
                    }
                  }
                  frame #2 {
                    n136 = call <userlib>:"Obtain Message Queue.vi"("name (unnamed)"="继保.vi") -> ("Message Queue"=w238:refnum<queue>)  [unwired: 9 in, 1 out]
                    n137 = Bundle(u16 257, TRUE) -> (w234:cluster{u16, bool})  [unwired: 1 in]
                    n138 = call-poly <userlib>:"Enqueue Message.vi"("Message Data"=w234, "Message"="遥控", "Message Queue"=w238) -> ()  [unwired: 7 in, 2 out]
                  }
                }
              }
            }
          }
        }
        n139 = call "报警更新.vi"("Message Data"=w183, "state"="动作更新") -> ()  [unwired: 10 in]
      }
      event "236": Value Change {
        n140 = event-data() -> ("CtlRef"=w239:refnum<vi>, "NewVal"=w240:bool)  [unwired: 1 in, 4 out]
        n141 = local read "整流柜远程/本地"() -> (w241:enum16{"零位", "本地", "远方"})
        n142 = case shown="真" w240 {
          selector: w240 -> [w243 w260]
          tunnel: w241 -> [w244 w261]
          tunnel: w239 -> [_ w258]
          frame False {
            n143 = case shown="\"远方\"" w244 {
              tunnel: w243 -> [w245 w249 _]
              frame "零位" {
                n144 = Not(x=w245) -> (.not. x?=w246:bool)
                n145 = local write "236"(w246) -> ()
                n146 = One Button Dialog(message="该权限在本地，不可投" ("消息")) -> ()  [unwired: 1 in, 1 out]
              }
              frame "本地", Default {
                n147 = Not(x=w249) -> (.not. x?=w248:bool)
                n148 = local write "236"(w248) -> ()
                n149 = One Button Dialog(message="该权限在本地，不可投" ("消息")) -> ()  [unwired: 1 in, 1 out]
              }
              frame "远方" {
                n150 = stacked-sequence {
                  frame #0 {
                    n151 = shared-variable "我的电脑\\PLC1200.lvlib\\40fromHMI模拟框架电流故障"(TRUE) -> ()  [unwired: 1 in, 1 out]
                  }
                  frame #1 {
                    n152 = Wait (ms)(milliseconds to wait=u32 30 ("等待时间（毫秒）")) -> ()  [unwired: 1 out]
                  }
                  frame #2 {
                    n153 = shared-variable "我的电脑\\PLC1200.lvlib\\40fromHMI模拟框架电流故障"(FALSE) -> ()  [unwired: 1 in, 1 out]
                  }
                  frame #3 {
                    n154 = Wait (ms)(milliseconds to wait=u32 30 ("等待时间（毫秒）")) -> ()  [unwired: 1 out]
                  }
                  frame #4 {
                    n155 = shared-variable "我的电脑\\PLC1200.lvlib\\40fromHMI故障复位"(TRUE) -> ()  [unwired: 1 in, 1 out]
                  }
                  frame #5 {
                    n156 = Wait (ms)(milliseconds to wait=u32 30 ("等待时间（毫秒）")) -> ()  [unwired: 1 out]
                  }
                  frame #6 {
                    n157 = shared-variable "我的电脑\\PLC1200.lvlib\\40fromHMI故障复位"(FALSE) -> ()  [unwired: 1 in, 1 out]
                  }
                }
              }
            }
          }
          frame True {
            n158 = local read "236-7"() -> (w259:bool)
            n159 = case shown="真" w259 {
              tunnel: w261 -> [w263 _]
              tunnel: w260 -> [w262 _]
              tunnel: w258 -> [_ w277]
              frame False {
                n160 = case shown="\"远方\"" w263 {
                  tunnel: w262 -> [w264 w267 w270]
                  frame "零位" {
                    n161 = Not(x=w264) -> (.not. x?=w265:bool)
                    n162 = local write "236"(w265) -> ()
                    n163 = One Button Dialog(message="该权限在本地，不可投" ("消息")) -> ()  [unwired: 1 in, 1 out]
                  }
                  frame "本地", Default {
                    n164 = Not(x=w267) -> (.not. x?=w268:bool)
                    n165 = local write "236"(w268) -> ()
                    n166 = One Button Dialog(message="该权限在本地，不可投" ("消息")) -> ()  [unwired: 1 in, 1 out]
                  }
                  frame "远方" {
                    n167 = stacked-sequence {
                      tunnel: w270 -> [_ _ _]
                      frame #0 {
                        n168 = shared-variable "我的电脑\\PLC1200.lvlib\\10fromHMI模拟中压合闸"(TRUE) -> ()  [unwired: 1 in, 1 out]
                      }
                      frame #1 {
                        n169 = Wait (ms)(milliseconds to wait=u32 30 ("等待时间（毫秒）")) -> ()  [unwired: 1 out]
                      }
                      frame #2 {
                        n170 = shared-variable "我的电脑\\PLC1200.lvlib\\10fromHMI模拟中压合闸"(FALSE ("10fromHMI模拟中压合闸")) -> ()  [unwired: 1 in, 1 out]
                      }
                    }
                    n171 = call "报警更新.vi"("Message Data"="整流柜远方>模拟中亚合闸" ("字符串"), "state"="动作更新") -> ()  [unwired: 10 in]
                  }
                }
              }
              frame True {
                n172 = property class="Bool (严格)"(reference=w277, "Value"=FALSE ("值")) -> ()  [unwired: 1 in, 2 out]
              }
            }
          }
        }
      }
      event "236-7", "237-7", "231-7", "241-7", "237": Value Change {
        n173 = event-data() -> ("CtlRef"=w281:refnum<vi>)  [unwired: 1 in]
        n174 = property class="Bool (严格)"(reference=w281) -> (reference out=w278:refnum<vi>, "Label.Text"=w280:string, "Value"=w279:T1)  [unwired: 1 in, 1 out]
        n175 = case shown="\"237-7\"" w280 {
          tunnel: w279 -> [_ w284 w290 w296 w302 w308 w314 w320]
          tunnel: w278 -> [_ w283 w289 w295 w301 w307 w313 w319]
          frame "假", Default {
          }
          frame "236-7" {
            n176 = case shown="真" w284 {
              tunnel: w283 -> [_ w286]
              frame False {
              }
              frame True {
                n177 = local read "236"() -> (w285:bool)
                n178 = case shown="真" w285 {
                  tunnel: w286 -> [_ w288]
                  frame False {
                  }
                  frame True {
                    n179 = property class="Bool (严格)"(reference=w288, "Value"=T1 FALSE ("值")) -> ()  [unwired: 1 in, 2 out]
                  }
                }
              }
            }
          }
          frame "237-7" {
            n180 = case shown="真" w290 {
              tunnel: w289 -> [_ w292]
              frame False {
              }
              frame True {
                n181 = local read "237"() -> (w291:bool)
                n182 = case shown="真" w291 {
                  tunnel: w292 -> [_ w294]
                  frame False {
                  }
                  frame True {
                    n183 = property class="Bool (严格)"(reference=w294, "Value"=T1 FALSE ("值")) -> ()  [unwired: 1 in, 2 out]
                  }
                }
              }
            }
          }
          frame "231-7" {
            n184 = case shown="真" w296 {
              tunnel: w295 -> [_ w298]
              frame False {
              }
              frame True {
                n185 = local read "231"() -> (w297:T1)
                n186 = case shown="真" w297 {
                  tunnel: w298 -> [_ w300]
                  frame False {
                  }
                  frame True {
                    n187 = property class="Bool (严格)"(reference=w300, "Value"=T1 FALSE ("值")) -> ()  [unwired: 1 in, 2 out]
                  }
                }
              }
            }
          }
          frame "241-7" {
            n188 = case shown="真" w302 {
              tunnel: w301 -> [_ w304]
              frame False {
              }
              frame True {
                n189 = local read "241"() -> (w303:T1)
                n190 = case shown="真" w303 {
                  tunnel: w304 -> [_ w306]
                  frame False {
                  }
                  frame True {
                    n191 = property class="Bool (严格)"(reference=w306, "Value"=T1 FALSE ("值")) -> ()  [unwired: 1 in, 2 out]
                  }
                }
              }
            }
          }
          frame "237" {
            n192 = case shown="真" w308 {
              tunnel: w307 -> [_ w310]
              frame False {
              }
              frame True {
                n193 = local read "237-7"() -> (w309:bool)
                n194 = case shown="真" w309 {
                  tunnel: w310 -> [_ w312]
                  frame False {
                  }
                  frame True {
                    n195 = property class="Bool (严格)"(reference=w312, "Value"=T1 FALSE ("值")) -> ()  [unwired: 1 in, 2 out]
                  }
                }
              }
            }
          }
          frame "231" {
            n196 = case shown="真" w314 {
              tunnel: w313 -> [_ w316]
              frame False {
              }
              frame True {
                n197 = local read "231-7"() -> (w315:bool)
                n198 = case shown="真" w315 {
                  tunnel: w316 -> [_ w318]
                  frame False {
                  }
                  frame True {
                    n199 = property class="Bool (严格)"(reference=w318, "Value"=T1 FALSE ("值")) -> ()  [unwired: 1 in, 2 out]
                  }
                }
              }
            }
          }
          frame "241" {
            n200 = case shown="真" w320 {
              tunnel: w319 -> [_ w322]
              frame False {
              }
              frame True {
                n201 = local read "241-7"() -> (w321:bool)
                n202 = case shown="真" w321 {
                  tunnel: w322 -> [_ w324]
                  frame False {
                  }
                  frame True {
                    n203 = property class="Bool (严格)"(reference=w324, "Value"=T1 FALSE ("值")) -> ()  [unwired: 1 in, 2 out]
                  }
                }
              }
            }
          }
        }
      }
      event Panel Close? {
        # "Send the 'Confirm Quit' message if the user closes the panel of the VI. Discard the event so the 'Confirm Quit' message has a chance to run."
        n204 = event-data() -> ()  [unwired: 1 in, 1 out]
        n205 = call-poly <userlib>:"Enqueue Message.vi"("Priority Message? (F)"=TRUE, "Message"="Confirm Quit", "Message Queue"=w329) -> ("error out"=w328:errorcluster, "dup Message Queue"=w327:refnum<queue>)  [unwired: 7 in]
        n206 = event-data("Discard?"=TRUE) -> ()  [unwired: 1 in, 1 out]
      }
      event Application Instance Close {
        # "#CodeRecommended - When a project closes, all VIs within that project are aborted and leave memory. However, any code placed in this event frame is guaranteed to run to completion, so add any cleanup code that absolutely must happen here."
        n207 = event-data() -> ()  [unwired: 1 in, 1 out]
      }
      event User Event {
        # "The Message Handling Loop processed an \"Exit\" message, which fired this event to stop the Event Handling Loop."
        n208 = event-data() -> ()  [unwired: 1 in, 1 out]
      }
      event "Exit": Value Change {
        # "Exit all of the program,and do not change the Box"
        n209 = event-data() -> ()  [unwired: 1 in, 1 out]
        n210 = call-poly <userlib>:"Enqueue Message.vi"("Priority Message? (F)"=TRUE, "Message"="Confirm Quit", "Message Queue"=w338) -> ("error out"=w336:errorcluster, "dup Message Queue"=w337:refnum<queue>)  [unwired: 7 in]
      }
    }
    n211 = call <userlib>:"Error Handler - Event Handling Loop.vi"("error in (no error)"=w28, "Message Queue"=w26) -> ("dup error in"=w25:errorcluster)  [unwired: 8 in, 1 out]
  }
  n212 = while {
    tunnel: w7 -> [w342]
    shift-right: [w349] -> _
    shift-left: w12 -> [w350]
    tunnel: w18 -> [w347]
    tunnel: w22 -> [w346]
    tunnel: [w340] -> w21
    stop <- w348 stop-if-true
    # "Comsumer Loop"
    n213 = call <userlib>:"Dequeue Message.vi"("error in (no error)"=w346, "Message Queue"=w342) -> ("error out"=w345:errorcluster, "Message Data"=w343:variant, "Message"=w344:string, "dup Message Queue"=w341:refnum<queue>)  [unwired: 6 in]
    n214 = case "Message Cases" shown="\"Initialize1\"" w344 {
      tunnel: w341 -> [_ w360 _ w377 w385 _ _ _ _ _ _ _ w469 w492 w508 w548 w570 w608 w632 _ _ _ _ _]
      tunnel: w345 -> [w351 w355 w374 w381 w390 w435 w446 w448 w450 w451 w454 w456 w487 w504 w512 w550 w574 w612 w635 w675 w688 w706 w722 w729]
      tunnel: [w351 w356 w369 w379 w390 w435 w446 w448 w450 w451 w454 w456 w487 w504 w512 w550 w574 w612 w635 w675 w688 w706 w722 w729] -> w339
      tunnel: w350 -> [w352 w359 w366 w380 w388 w420 w441 w447 w449 w452 w453 w455 w478 w503 w507 w549 w573 w611 w634 w674 w687 w705 w721 w728]
      tunnel: [w352 w359 w366 w380 w387 w391 w441 w447 w449 w452 w453 w455 w464 w503 w507 w549 w573 w611 w634 w674 w687 w705 w721 w728] -> w349
      tunnel: [_ TRUE _ _ _ _ _ _ _ _ _ _ _ _ _ _ _ _ _ _ _ _ _ _] -> w348
      tunnel: w343 -> [_ _ w373 _ _ _ _ _ _ _ _ _ _ _ _ _ _ _ _ w652 w685 w703 w719 _]
      tunnel: w347 -> [_ w354 _ _ _ _ _ _ _ _ _ _ _ _ _ _ _ _ _ _ _ _ _ _]
      frame Default {
        # "'Default' case only runs if there is a message that isn't defined in any of the other cases.  Output a programming error."
      }
      frame "Exit" {
        # "Stop the VI"
        # "Release the message queue reference"
        # "#CodeNeeded - Add any required cleanup code here"
        # "Exit - Exit the application."
        n215 = call <userlib>:"Fire User Event - Stop.vi"("User Event - Stop"=w354) -> ("error out"=w353:errorcluster)  [unwired: 10 in]
        n216 = Release Queue(queue=w360, error in (no error)=w355) -> (error out=w357:errorcluster)  [unwired: 1 in, 2 out]
        n217 = Merge Errors(w353, w357) -> (w356:errorcluster)
      }
      frame "Error" {
        # "Error - Check the error message data and respond accordingly. This message is sent by the \"Error Handler\" VIs at the end of each loop in this application."
        n218 = Unbundle By Name(w366) -> ("Thread.HostQ"=w365:string)
        n219 = Variant To Data(error in=w374, type=errorcluster {"status"=FALSE, "code"=0, "source"=""} ("error constant"), Variant=w373) -> (data=w362:errorcluster, error out=w371:errorcluster)
        n220 = To Variant(anything=w362) -> (Variant=w361:variant)
        n221 = call <userlib>:"Obtain Message Queue.vi"("name (unnamed)"=w365) -> ("error out"=w364:errorcluster, "Message Queue"=w363:refnum<queue>)  [unwired: 9 in]
        n222 = call-poly <userlib>:"Enqueue Message.vi"("Priority Message? (F)"=TRUE, "error in (no error)"=w364, "Message Data"=w361, "Message"="Error", "Message Queue"=w363) -> ("error out"=w370:errorcluster)  [unwired: 5 in, 1 out]
        n223 = Merge Errors(w370, w371) -> (w369:errorcluster)
      }
      frame "Confirm Quit" {
        # "#CodeNeeded - If you want to provide an \"Are you sure\" dialog (or some other notification) before the application exits, place that code here. This message is typically sent from a Panel Close? event."
        # "Confirm Quit - Message that can confirm whether or not the user wants to exit the application."
        n224 = call-poly <userlib>:"Enqueue Message.vi"("Priority Message? (F)"=TRUE, "error in (no error)"=w381, "Message"="Exit", "Message Queue"=w377) -> ("error out"=w378:errorcluster)  [unwired: 6 in, 1 out]
        n225 = Merge Errors(w378) -> (w379:errorcluster)
      }
      frame "Initialize" {
        # "Initialize - Send separate messages to initialize the data and the front panel.  Bundle control references."
        n226 = Unbundle By Name(w388) -> ("Thread.ThisVI"=w389:refnum<vi>)
        n227 = invoke class="VI" method="Default Vals.Reinit All"(reference=w389) -> ()  [unwired: 2 in, 3 out]
        n228 = call <userlib>:"Obtain Message Queue.vi"("name (unnamed)"="灯组解析.vi") -> ("Message Queue"=w382:refnum<queue>)  [unwired: 9 in, 1 out]
        n229 = call-poly <userlib>:"Enqueue Message.vi"("Message Array"=string[] ["Initialize1", "SendRef", "远方本地采集"] ("Message"), "Message Queue"=w385) -> ()  [unwired: 8 in, 2 out]
        n230 = Bundle By Name(cluster=w388, "远程本地"=T8 {"整流柜远程/本地"=enum."零位", "进线柜远程/本地"=enum."零位", "馈线柜远程/本地"=enum."零位", "负极柜远程/本地"=enum."零位", "上网柜远程/本地"=enum."零位", "直流继保远程/本地"=enum."零位"}, "Message Queue"=w382) -> (w387:T2)
      }
      frame "Initialize1" {
        n231 = control-ref of="225"() -> (w434:refnum<vi>)
        n232 = control-ref of="201"() -> (w433:refnum<vi>)
        n233 = control-ref of="202"() -> (w432:refnum<vi>)
        n234 = control-ref of="226"() -> (w431:refnum<vi>)
        n235 = control-ref of="236"() -> (w430:refnum<vi>)
        n236 = control-ref of="236-7"() -> (w429:refnum<vi>)
        n237 = control-ref of="237"() -> (w428:refnum<vi>)
        n238 = control-ref of="237-7"() -> (w427:refnum<vi>)
        n239 = control-ref of="231"() -> (w426:refnum<vi>)
        n240 = control-ref of="231-7"() -> (w425:refnum<vi>)
        n241 = control-ref of="245"() -> (w424:refnum<vi>)
        n242 = control-ref of="2451"() -> (w423:refnum<vi>)
        n243 = control-ref of="241"() -> (w422:refnum<vi>)
        n244 = control-ref of="241-7"() -> (w421:refnum<vi>)
        n245 = Bundle By Name(cluster=w420, "1-1.225"=w434, "1-1.201"=w433, "1-1.202"=w432, "1-1.226"=w431, "1-1.236"=w430, "1-1.236-7"=w429, "1-1.237"=w428, "1-1.237-7"=w427, "1-1.231"=w426, "1-1.231-7"=w425, "1-1.245"=w424, "1-1.2451"=w423, "1-1.241"=w422, "1-1.241-7"=w421) -> (w419:T2)
        n246 = control-ref of="60"() -> (w418:refnum<vi>)
        n247 = control-ref of="70"() -> (w417:refnum<vi>)
        n248 = control-ref of="2120"() -> (w416:refnum<vi>)
        n249 = control-ref of="212"() -> (w415:refnum<vi>)
        n250 = control-ref of="2121"() -> (w414:refnum<vi>)
        n251 = control-ref of="2124"() -> (w413:refnum<vi>)
        n252 = control-ref of="214"() -> (w412:refnum<vi>)
        n253 = control-ref of="2140"() -> (w411:refnum<vi>)
        n254 = control-ref of="2141"() -> (w410:refnum<vi>)
        n255 = control-ref of="90"() -> (w409:refnum<vi>)
        n256 = control-ref of="2110"() -> (w408:refnum<vi>)
        n257 = control-ref of="211"() -> (w407:refnum<vi>)
        n258 = control-ref of="2111"() -> (w406:refnum<vi>)
        n259 = control-ref of="2113"() -> (w405:refnum<vi>)
        n260 = Bundle By Name(cluster=w419, "1-2.60"=w418, "1-2.70"=w417, "1-2.2120"=w416, "1-2.212"=w415, "1-2.2121"=w414, "1-2.2124"=w413, "1-2.214"=w412, "1-2.2140"=w411, "1-2.2141"=w410, "1-2.90"=w409, "1-2.2110"=w408, "1-2.211"=w407, "1-2.2111"=w406, "1-2.2113"=w405) -> (w404:T2)
        n261 = control-ref of="65"() -> (w403:refnum<vi>)
        n262 = control-ref of="75"() -> (w402:refnum<vi>)
        n263 = control-ref of="401"() -> (w401:refnum<vi>)
        n264 = control-ref of="402"() -> (w400:refnum<vi>)
        n265 = control-ref of="445"() -> (w399:refnum<vi>)
        n266 = control-ref of="404"() -> (w398:refnum<vi>)
        n267 = control-ref of="213"() -> (w397:refnum<vi>)
        n268 = control-ref of="2130"() -> (w396:refnum<vi>)
        n269 = control-ref of="2131"() -> (w395:refnum<vi>)
        n270 = control-ref of="405"() -> (w394:refnum<vi>)
        n271 = control-ref of="406"() -> (w393:refnum<vi>)
        n272 = control-ref of="407"() -> (w392:refnum<vi>)
        n273 = Bundle By Name(cluster=w404, "2.65"=w403, "2.75"=w402, "2.401"=w401, "2.402"=w400, "2.445"=w399, "2.404"=w398, "2.213"=w397, "2.2130"=w396, "2.2131"=w395, "2.405"=w394, "2.406"=w393, "2.407"=w392) -> (w391:T2)
      }
      frame "SendRef" {
        (unwired) T10 {"1-1"={"225"=refnum, "201"=refnum, "202"=refnum, "226"=refnum, "236"=refnum, "236-7"=refnum, "237"=refnum, "237-7"=refnum, "231"=refnum, "231-7"=refnum, "245"=refnum, "2451"=refnum, "241"=refnum, "241-7"=refnum}, "1-2"={"60"=refnum, "70"=refnum, "2120"=refnum, "212"=refnum, "2121"=refnum, "2124"=refnum, "214"=refnum, "2140"=refnum, "2141"=refnum, "90"=refnum, "2110"=refnum, "211"=refnum, "2111"=refnum, "2113"=refnum}, "2"={"65"=refnum, "75"=refnum, "401"=refnum, "402"=refnum, "445"=refnum, "404"=refnum, "213"=refnum, "2130"=refnum, "2131"=refnum, "405"=refnum, "406"=refnum, "407"=refnum}} ("输出簇")
        n274 = Unbundle By Name(w441) -> ("1-1"=w440:T11, "1-2"=w439:T12, "2"=w438:T13)
        n275 = Bundle("1-1"=w440, "1-2"=w439, "2"=w438) -> (w437:T10)  [unwired: 1 in]
        n276 = call <userlib>:"Obtain Message Queue.vi"("name (unnamed)"="灯组解析.vi") -> ("error out"=w442:errorcluster, "Message Queue"=w445:refnum<queue>)  [unwired: 9 in]
        n277 = call-poly <userlib>:"Enqueue Message.vi"("Priority Message? (F)"=TRUE, "error in (no error)"=w442, "Message Data"=w437, "Message"="接收Ref" ("字符串"), "Message Queue"=w445) -> ()  [unwired: 5 in, 2 out]
      }
      frame "<-------UI-------->" {
      }
      frame "<------Core------>" {
      }
      frame "Core_InitializeRef" {
        # "Initialize control references. For there is not enough space to locate all the control references, separate the codes into 2 messages"
      }
      frame "<---Operation--->" {
      }
      frame "<------LOOP----->" {
      }
      frame "远方本地采集" {
        n278 = global read "global-opc.vi" "IP10"() -> (w486:T14)
        n279 = global read "global-opc.vi" "IP30"() -> (w484:T7)
        n280 = global read "global-opc.vi" "IP40"() -> (w483:T15)
        n281 = global read "global-opc.vi" "IP50"() -> (w482:T6)
        n282 = global read "global-2.vi" "开入"() -> (w462:T16)
        n283 = global read "global-opc.vi" "IP20"() -> (w485:T17)
        n284 = Unbundle By Name(w484) -> ("toHMI远方"=w475:bool, "toHMI本地"=w474:bool)
        n285 = Unbundle By Name(w483) -> ("toHMI远程"=w473:bool, "toHMI本地"=w472:bool)
        n286 = Unbundle By Name(w486) -> ("toHMI远程"=w481:bool, "toHMI本地"=w480:bool)
        n287 = Unbundle By Name(w485) -> ("toHMI远程"=w476:bool, "toHMI本地"=w477:bool)
        n288 = Unbundle By Name(w482) -> ("toHMI远程"=w471:bool, "toHMI本地"=w461:bool)
        n289 = Unbundle By Name(w462) -> ("远程控制"=w460:bool, "就地控制"=w459:bool)
        n290 = call-poly <userlib>:"Enqueue Message.vi"("Message"="本地远程条件判断", "Message Queue"=w469) -> ("error out"=w457:errorcluster)  [unwired: 8 in, 1 out]
        n291 = call "远程本地判断.vi"("toHMI本地"=w472, "toHMI远程"=w473) -> ("远程/本地"=w466:enum16{"零位", "本地", "远方"})
        "负极柜远程/本地" <- w466
        n292 = call "远程本地判断.vi"("toHMI本地"=w461, "toHMI远程"=w471) -> ("远程/本地"=w465:enum16{"零位", "本地", "远方"})
        "上网柜远程/本地" <- w465
        n293 = call "远程本地判断.vi"("toHMI本地"=w459, "toHMI远程"=w460) -> ("远程/本地"=w458:enum16{"零位", "本地", "远方"})
        "直流继保远程/本地" <- w458
        n294 = call "远程本地判断.vi"("toHMI本地"=w474, "toHMI远程"=w475) -> ("远程/本地"=w467:enum16{"零位", "本地", "远方"})
        "馈线柜远程/本地" <- w467
        n295 = call "远程本地判断.vi"("toHMI本地"=w480, "toHMI远程"=w481) -> ("远程/本地"=w479:enum16{"零位", "本地", "远方"})
        "整流柜远程/本地" <- w479
        n296 = call "远程本地判断.vi"("toHMI本地"=w477, "toHMI远程"=w476) -> ("远程/本地"=w468:enum16{"零位", "本地", "远方"})
        "进线柜远程/本地" <- w468
        n297 = flat-sequence {
          tunnel: w457 -> [_]
          frame #0 {
            n298 = Wait (ms)(milliseconds to wait=u32 10 ("等待时间（毫秒）")) -> ()  [unwired: 1 out]
          }
        }
        n299 = Bundle By Name(cluster=w478, "远程本地.整流柜远程/本地"=w479, "远程本地.进线柜远程/本地"=w468, "远程本地.馈线柜远程/本地"=w467, "远程本地.负极柜远程/本地"=w466, "远程本地.上网柜远程/本地"=w465, "远程本地.直流继保远程/本地"=w458) -> (w464:T2)
        n300 = Unbundle By Name(w464) -> ("远程本地"=w463:T8)
        n301 = global write "远程本地T.vi" "远程本地"(w463) -> ()
      }
      frame "本地远程条件判断" {
        n302 = call-poly <userlib>:"Enqueue Message.vi"("Message"="整流柜远程本地", "Message Queue"=w492) -> ()  [unwired: 8 in, 2 out]
        n303 = global read "global-opc.vi" "IP10"() -> (w502:T14)
        n304 = global read "global-opc.vi" "IP20"() -> (w501:T17)
        n305 = global read "global-opc.vi" "IP30"() -> (w500:T7)
        n306 = global read "global-opc.vi" "IP50"() -> (w499:T6)
        n307 = Unbundle By Name(w501) -> ("toHMI远程"=w496:bool)
        n308 = Unbundle By Name(w500) -> ("toHMI远方"=w489:bool)
        n309 = Unbundle By Name(w499) -> ("toHMI远程"=w494:bool)
        n310 = Unbundle By Name(w502) -> ("toHMI远程"=w498:bool)
        n311 = call "条件禁用.vi"("远程"=w496, "state"="直流进线柜BOOL", "队列输入"=w492) -> ()  [unwired: 9 in]
        n312 = call "条件禁用.vi"("远程"=w498, "state"="整流器柜BOOL", "队列输入"=w492) -> ()  [unwired: 9 in]
        n313 = call "条件禁用.vi"("远程"=w489, "state"="直流馈线柜BOOL", "队列输入"=w492) -> ()  [unwired: 9 in]
        n314 = call "条件禁用.vi"("远程"=w494, "state"="上网柜BOOL", "队列输入"=w492) -> ()  [unwired: 9 in]
      }
      frame "整流柜远程本地" {
        n315 = Unbundle By Name(w507) -> ("远程本地.整流柜远程/本地"=w511:enum16{"零位", "本地", "远方"}, "Message Queue"=w506:refnum<queue>)
        "整流柜远程/本地" <- w511
        n316 = global read "global-opc.vi" "IP10"() -> (w510:T14)
        n317 = call-poly <userlib>:"Enqueue Message.vi"("Message"="负极柜远程本地", "Message Queue"=w508) -> ()  [unwired: 8 in, 2 out]
        n318 = First Call?() -> (First Call?: T/F=w505:bool)
        n319 = case shown="假" w505 {
          tunnel: w511 -> [w515 _]
          tunnel: w510 -> [w514 w536]
          tunnel: w506 -> [w513 w535]
          frame False {
            n320 = case shown="\"本地\"" w515 {
              tunnel: w514 -> [_ w524 w533]
              tunnel: w513 -> [_ w521 w531]
              frame "零位", Default {
              }
              frame "本地" {
                n321 = Unbundle By Name(w524) -> ("toHMI模拟中压合闸—按钮"=w522:bool)
                n322 = call "下降沿.vi"("Boolean Input"=w522) -> ("Falling Edge"=w520:bool)
                n323 = call "上升沿.vi"("Boolean Input"=w522) -> ("Rising Edge"=w523:bool)
                n324 = call "send-loop.vi"("set"=bool[] [TRUE, TRUE, TRUE, TRUE, TRUE, TRUE, TRUE, TRUE], "loop"=string[] ["201", "202", "225", "226", "236", "237", "231", "241"], "case-in"=w523, "队列输入"=w521) -> ()  [unwired: 7 in, 1 out]
                n325 = call "send-loop.vi"("set"=bool[] [TRUE, TRUE], "loop"=string[] ["236", "237"], "case-in"=w520, "队列输入"=w521) -> ()  [unwired: 7 in, 1 out]
              }
              frame "远方" {
                n326 = Unbundle By Name(w533) -> ("toHMI模拟中压合闸—按钮"=w530:bool)
                n327 = call "上升沿.vi"("Boolean Input"=w530) -> ("Rising Edge"=w532:bool)
                n328 = call "下降沿.vi"("Boolean Input"=w530) -> ("Falling Edge"=w529:bool)
                n329 = call "send-loop.vi"("set"=bool[] [TRUE, TRUE, TRUE, TRUE, TRUE, TRUE, TRUE, TRUE], "loop"=string[] ["201", "202", "225", "226", "236", "237", "231", "241"], "case-in"=w532, "队列输入"=w531) -> ()  [unwired: 7 in, 1 out]
                n330 = call "send-loop.vi"("set"=bool[] [TRUE, TRUE], "loop"=string[] ["236", "237"], "case-in"=w529, "队列输入"=w531) -> ()  [unwired: 7 in, 1 out]
              }
            }
          }
          frame True {
            n331 = Unbundle By Name(w536) -> ("toHMI模拟中压合闸—按钮"=w534:bool)
            n332 = case shown="真" w534 {
              tunnel: w535 -> [_ w540]
              tunnel: w534 -> [_ w539]
              frame False {
              }
              frame True {
                w538 = string[] ["201", "202", "225", "226", "2451", "245", "236", "237", "231", "241", "401", "402", "445", "404", "405", "406", "407"]
                n333 = for {
                  tunnel: w538 -> [_] mode=indexing
                  tunnel: [TRUE] -> w537 mode=indexing
                }
                n334 = call "send-loop.vi"("set"=w537, "loop"=w538, "case-in"=w539, "队列输入"=w540) -> ()  [unwired: 7 in, 1 out]
              }
            }
          }
        }
      }
      frame "进线柜远程本地" {
        n335 = Unbundle By Name(w549) -> ("Message Queue"=w543:refnum<queue>)
        n336 = call-poly <userlib>:"Enqueue Message.vi"("Message"="馈线柜远程本地", "Message Queue"=w548) -> ()  [unwired: 8 in, 2 out]
        n337 = global read "global-opc.vi" "IP20"() -> (w546:T17)
        n338 = Unbundle By Name(w546) -> ("toHMI刀开关合—状态"=w544:bool, "toHMI刀开关分—状态"=w545:bool)
        n339 = First Call?() -> (First Call?: T/F=w542:bool)
        n340 = case shown="假" w542 {
          tunnel: w545 -> [w555 _]
          tunnel: w544 -> [w553 w559]
          tunnel: w543 -> [w551 w560]
          frame False {
            w557 = string[] ["60", "70", "90"]
            n341 = call "上升沿.vi"("Boolean Input"=w553) -> ("Rising Edge"=w552:bool)
            n342 = call "上升沿.vi"("Boolean Input"=w555) -> ("Rising Edge"=w554:bool)
            n343 = call "send-loop.vi"("set"=bool[] [TRUE, TRUE, TRUE], "loop"=w557, "case-in"=w552, "队列输入"=w551) -> ()  [unwired: 7 in, 1 out]
            n344 = call "send-loop.vi"("set"=bool[] [FALSE, FALSE, FALSE], "loop"=w557, "case-in"=w554, "队列输入"=w551) -> ()  [unwired: 7 in, 1 out]
          }
          frame True {
            n345 = case shown="真" w559 {
              selector: w559 -> [_ w561]
              tunnel: w560 -> [_ w562]
              frame False {
              }
              frame True {
                n346 = call "send-loop.vi"("set"=bool[] [TRUE, TRUE, TRUE], "loop"=string[] ["60", "70", "90"], "case-in"=w561, "队列输入"=w562) -> ()  [unwired: 7 in, 1 out]
              }
            }
          }
        }
      }
      frame "馈线柜远程本地" {
        n347 = Unbundle By Name(w573) -> ("Message Queue"=w567:refnum<queue>)
        n348 = global read "global-opc.vi" "IP30"() -> (w572:T7)
        n349 = Unbundle By Name(w572) -> ("toHMI高断合—状态"=w568:bool, "toHMI高断分—状态"=w569:bool, "toHMI旁路合分闸—状态"=w565:bool)
        n350 = call-poly <userlib>:"Enqueue Message.vi"("Message"="上网柜远程本地", "Message Queue"=w570) -> ()  [unwired: 8 in, 2 out]
        n351 = First Call?() -> (First Call?: T/F=w566:bool)
        n352 = case shown="假" w566 {
          tunnel: w569 -> [w587 _]
          tunnel: w568 -> [w585 w594]
          tunnel: w567 -> [w583 w592]
          tunnel: w565 -> [w576 w593]
          frame False {
            w575 = string[] ["2120", "2140", "2110", "2130"]
            w589 = string[] ["212", "214", "211", "213"]
            n353 = call "上升沿.vi"("Boolean Input"=w585) -> ("Rising Edge"=w584:bool)
            n354 = call "上升沿.vi"("Boolean Input"=w587) -> ("Rising Edge"=w586:bool)
            n355 = call "send-loop.vi"("set"=bool[] [TRUE, TRUE, TRUE, TRUE, FALSE], "loop"=w589, "case-in"=w584, "队列输入"=w583) -> ()  [unwired: 7 in, 1 out]
            n356 = call "send-loop.vi"("set"=bool[] [FALSE, FALSE, FALSE, FALSE], "loop"=w589, "case-in"=w586, "队列输入"=w583) -> ("dup Message Queue"=w578:refnum<queue>)  [unwired: 7 in]
            n357 = call "下降沿.vi"("Boolean Input"=w576) -> ("Falling Edge"=w581:bool)
            n358 = call "上升沿.vi"("Boolean Input"=w576) -> ("Rising Edge"=w579:bool)
            n359 = call "send-loop.vi"("set"=bool[] [TRUE, TRUE, TRUE, TRUE], "loop"=w575, "case-in"=w579, "队列输入"=w578) -> ("dup Message Queue"=w577:refnum<queue>)  [unwired: 7 in]
            n360 = call "send-loop.vi"("set"=bool[] [FALSE, FALSE, FALSE, FALSE], "loop"=w575, "case-in"=w581, "队列输入"=w577) -> ()  [unwired: 7 in, 1 out]
          }
          frame True {
            n361 = case shown="真" w594 {
              selector: w594 -> [_ w601]
              tunnel: w592 -> [w599 w600]
              tunnel: [w599 w600] -> w591
              frame False {
              }
              frame True {
                n362 = call "send-loop.vi"("set"=bool[] [TRUE, TRUE, TRUE, TRUE, FALSE], "loop"=string[] ["212", "214", "211", "213"], "case-in"=w601, "队列输入"=w600) -> ()  [unwired: 7 in, 1 out]
              }
            }
            n363 = case shown="真" w593 {
              selector: w593 -> [_ w596]
              tunnel: w591 -> [_ w595]
              frame False {
              }
              frame True {
                n364 = call "send-loop.vi"("set"=bool[] [TRUE, TRUE, TRUE, TRUE], "loop"=string[] ["2120", "2140", "2110", "2130"], "case-in"=w596, "队列输入"=w595) -> ()  [unwired: 7 in, 1 out]
              }
            }
          }
        }
      }
      frame "负极柜远程本地" {
        n365 = global read "global-opc.vi" "IP40"() -> (w610:T15)
        n366 = Unbundle By Name(w610) -> ("toHMI刀开关合—状态"=w606:bool, "toHMI刀开关分—状态"=w605:bool)
        n367 = Unbundle By Name(w611) -> ("Message Queue"=w607:refnum<queue>)
        n368 = call-poly <userlib>:"Enqueue Message.vi"("Message"="进线柜远程本地", "Message Queue"=w608) -> ()  [unwired: 8 in, 2 out]
        n369 = First Call?() -> (First Call?: T/F=w604:bool)
        n370 = case shown="真" w604 {
          tunnel: w607 -> [w620 w621]
          tunnel: w606 -> [w616 w622]
          tunnel: w605 -> [w614 _]
          frame False {
            w618 = string[] ["65", "75"]
            n371 = call "上升沿.vi"("Boolean Input"=w616) -> ("Rising Edge"=w615:bool)
            n372 = call "上升沿.vi"("Boolean Input"=w614) -> ("Rising Edge"=w613:bool)
            n373 = call "send-loop.vi"("set"=bool[] [FALSE, FALSE], "loop"=w618, "case-in"=w613, "队列输入"=w620) -> ()  [unwired: 7 in, 1 out]
            n374 = call "send-loop.vi"("set"=bool[] [TRUE, TRUE], "loop"=w618, "case-in"=w615, "队列输入"=w620) -> ()  [unwired: 7 in, 1 out]
          }
          frame True {
            n375 = case shown="真" w622 {
              selector: w622 -> [_ w623]
              tunnel: w621 -> [_ w624]
              frame False {
              }
              frame True {
                n376 = call "send-loop.vi"("set"=bool[] [TRUE, TRUE], "loop"=string[] ["65", "75"], "case-in"=w623, "队列输入"=w624) -> ()  [unwired: 7 in, 1 out]
              }
            }
          }
        }
      }
      frame "上网柜远程本地" {
        n377 = Unbundle By Name(w634) -> ("Message Queue"=w628:refnum<queue>)
        n378 = global read "global-opc.vi" "IP50"() -> (w631:T6)
        n379 = Unbundle By Name(w631) -> ("toHMI刀开关合—状态"=w630:bool, "toHMI刀开关分—状态"=w629:bool)
        n380 = call-poly <userlib>:"Enqueue Message.vi"("Message"="远方本地采集", "Message Queue"=w632) -> ()  [unwired: 8 in, 2 out]
        n381 = First Call?() -> (First Call?: T/F=w627:bool)
        n382 = case shown="真" w627 {
          tunnel: w630 -> [w643 w645]
          tunnel: w629 -> [w638 _]
          tunnel: w628 -> [w636 w644]
          frame False {
            w639 = string[] ["2121", "2141", "2124", "2111", "2131", "2113"]
            n383 = call "上升沿.vi"("Boolean Input"=w643) -> ("Rising Edge"=w642:bool)
            n384 = call "上升沿.vi"("Boolean Input"=w638) -> ("Rising Edge"=w637:bool)
            n385 = call "send-loop.vi"("set"=bool[] [TRUE, TRUE, TRUE, TRUE, TRUE, TRUE, TRUE, TRUE, TRUE], "loop"=w639, "case-in"=w642, "队列输入"=w636) -> ()  [unwired: 7 in, 1 out]
            n386 = call "send-loop.vi"("set"=bool[] [FALSE, FALSE, FALSE, FALSE, FALSE, FALSE, FALSE, FALSE, FALSE], "loop"=w639, "case-in"=w637, "队列输入"=w636) -> ()  [unwired: 7 in, 1 out]
          }
          frame True {
            n387 = case shown="真" w645 {
              selector: w645 -> [_ w648]
              tunnel: w644 -> [_ w649]
              frame False {
              }
              frame True {
                n388 = call "send-loop.vi"("set"=bool[] [TRUE, TRUE, TRUE, TRUE, TRUE, TRUE, TRUE, TRUE, TRUE], "loop"=string[] ["2121", "2141", "2124", "2111", "2131", "2113"], "case-in"=w648, "队列输入"=w649) -> ()  [unwired: 7 in, 1 out]
              }
            }
          }
        }
      }
      frame "整流器柜BOOL" {
        n389 = Unbundle By Name(w674) -> ("1-1.225"=w673:refnum<vi>, "1-1.201"=w672:refnum<vi>, "1-1.202"=w671:refnum<vi>, "1-1.226"=w670:refnum<vi>, "1-1.236-7"=w669:refnum<vi>, "1-1.237"=w668:refnum<vi>, "1-1.237-7"=w667:refnum<vi>, "1-1.231"=w666:refnum<vi>, "1-1.231-7"=w665:refnum<vi>, "1-1.245"=w664:refnum<vi>, "1-1.2451"=w663:refnum<vi>, "1-1.241"=w662:refnum<vi>, "1-1.241-7"=w661:refnum<vi>, "2.401"=w660:refnum<vi>, "2.402"=w659:refnum<vi>, "2.445"=w658:refnum<vi>, "2.404"=w657:refnum<vi>, "2.405"=w656:refnum<vi>, "2.406"=w655:refnum<vi>, "2.407"=w654:refnum<vi>)
        n390 = Variant To Data(type=FALSE, Variant=w652) -> (data=w650:bool)  [unwired: 1 in, 1 out]
        n391 = Build Array(w673, w672, w671, w670, w669, w668, w667, w666, w665, w664, w663, w662, w661, w660, w659, w658, w657, w656, w655, w654) -> (w653:refnum<vi>[])
        n392 = for {
          tunnel: w653 -> [w680] mode=indexing
          tunnel: w650 -> [w676]
          n393 = Select(t=T9."Enabled" ("禁用"), s=w676, f=T9."Disabled" ("禁用")) -> (s? t:f=w678:T9)
          n394 = property class="Bool (严格)"(reference=w680, "DisabledEnum"=w678) -> ()  [unwired: 1 in, 2 out]
        }
      }
      frame "直流进线柜BOOL" {
        n395 = Unbundle By Name(w687) -> ("1-2.70"=w682:refnum<vi>, "1-2.90"=w681:refnum<vi>)
        n396 = Variant To Data(type=FALSE, Variant=w685) -> (data=w683:bool)  [unwired: 1 in, 1 out]
        n397 = Build Array(w682, w681) -> (w686:refnum<vi>[])
        n398 = for {
          tunnel: w686 -> [w689] mode=indexing
          tunnel: w683 -> [w690]
          n399 = Select(t=T9."Enabled" ("禁用"), s=w690, f=T9."Disabled" ("禁用")) -> (s? t:f=w692:T9)
          n400 = property class="Bool (严格)"(reference=w689, "DisabledEnum"=w692) -> ()  [unwired: 1 in, 2 out]
        }
      }
      frame "直流馈线柜BOOL" {
        n401 = Unbundle By Name(w705) -> ("1-2.214"=w700:refnum<vi>, "1-2.211"=w699:refnum<vi>, "2.213"=w698:refnum<vi>, "1-2.2120"=w697:refnum<vi>, "1-2.2140"=w696:refnum<vi>, "1-2.2110"=w695:refnum<vi>, "2.2130"=w694:refnum<vi>)
        n402 = Variant To Data(type=FALSE, Variant=w703) -> (data=w701:bool)  [unwired: 1 in, 1 out]
        n403 = Build Array(w700, w699, w698, w697, w696, w695, w694) -> (w704:refnum<vi>[])
        n404 = for {
          tunnel: w704 -> [w707] mode=indexing
          tunnel: w701 -> [w708]
          n405 = Select(t=T9."Enabled" ("禁用"), s=w708, f=T9."Disabled" ("禁用")) -> (s? t:f=w710:T9)
          n406 = property class="Bool (严格)"(reference=w707, "DisabledEnum"=w710) -> ()  [unwired: 1 in, 2 out]
        }
      }
      frame "上网柜BOOL" {
        n407 = Unbundle By Name(w721) -> ("1-2.2124"=w716:refnum<vi>, "1-2.2141"=w715:refnum<vi>, "1-2.2111"=w714:refnum<vi>, "1-2.2113"=w713:refnum<vi>, "2.2131"=w712:refnum<vi>)
        n408 = Variant To Data(type=FALSE, Variant=w719) -> (data=w717:bool)  [unwired: 1 in, 1 out]
        n409 = Build Array(w716, w715, w714, w713, w712) -> (w720:refnum<vi>[])
        n410 = for {
          tunnel: w720 -> [w723] mode=indexing
          tunnel: w717 -> [w724]
          n411 = Select(t=T9."Enabled" ("禁用"), s=w724, f=T9."Disabled" ("禁用")) -> (s? t:f=w726:T9)
          n412 = property class="Bool (严格)"(reference=w723, "DisabledEnum"=w726) -> ()  [unwired: 1 in, 2 out]
        }
      }
      frame "212" {
      }
    }
    n413 = call <userlib>:"Error Handler - Message Handling Loop.vi"("error in (no error)"=w339, "Message Queue"=w341) -> ("dup error in"=w340:errorcluster)  [unwired: 8 in, 1 out]
  }
  n414 = Unregister For Events(event registration refnum=w16, error in=w15) -> (error out=w17:errorcluster)
  n415 = Merge Errors(w17, w21) -> (w19:errorcluster)
  n416 = call <userlib>:"Destroy User Event - Stop.vi"("error in (no error)"=w19, "User Event - Stop"=w18) -> ()  [unwired: 9 in, 1 out]
